vi "Save-Recall State.vi"(0 "VISA resource name":refnum<visa-resource-name>, 1 "saver's name":string, 2 "saved state comments":string, 5 "save/recall (f : recall)":bool, 7 "file name (read description)":path, 11 "error in (no error)":errorcluster, 12 "saved state title":string) -> (3 "recaller's name":string, 4 "VISA resource name out":refnum<visa-resource-name>, 6 "recalled state comments":string, 8 "recalled state date":string, 10 "recalled state time":string, 14 "recalled state title":string, 15 "error out":errorcluster)   [LabVIEW 2018, in "Agilent 87XX Series.lvlib"]
doc: "This VI for the HP8753B Network Analyzer is used for saving instrument states. An instrument state is all the stimulus and response parameters that set up the instrument to make a specific measurement. This information is called the learn string.\n\n The learn string is an encoded array containing only the data need to re-create the state. For example, to re-create a frequency list the HP8753B only needs to save the start frequency, frequency span, and the number of points in each segment. Each point is not recorded. Thus the size of the learn string is not proportional to the number of points in the sweep.\n\n To save calibration data and memory traces you must use the \"save/recall calibration\" and \"save/recall data\" VIs.\n\n When a state is recalled with this VI, the saver's name, the state title, and the save date are written to the instrument display."
uses:
  Agilent 87XX Series.lvlib
panel:
  # "save to file\nrecall from file"
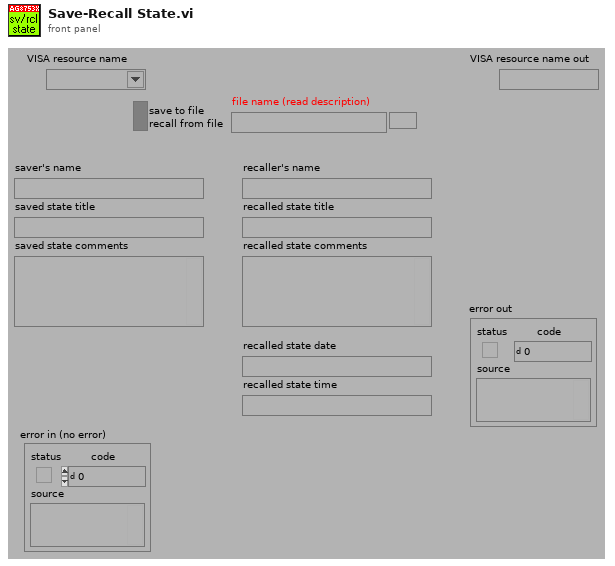
[diagram p1: front panel]
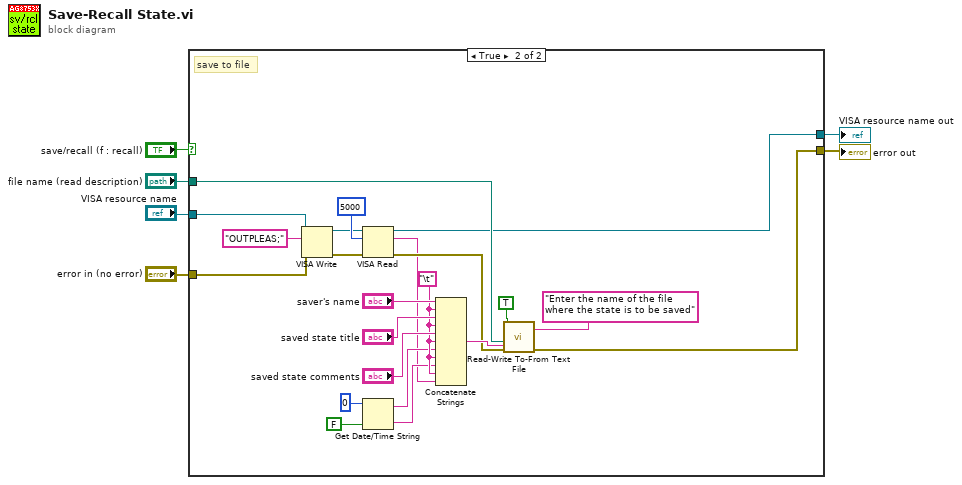
[diagram p0: block diagram]
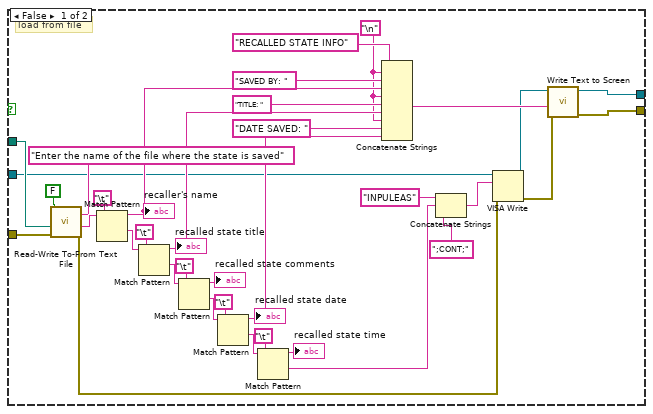
[diagram p2: hidden frame]
diagram:
  n1 = case shown="True" "save/recall (f : recall)" {
    tunnel: "VISA resource name" -> [w16 w50]
    tunnel: "file name (read description)" -> [w20 w51]
    tunnel: "error in (no error)" -> [w15 w49]
    tunnel: [w10 w45] -> w2
    tunnel: [w9 w46] -> w1
    frame False {
      w23 = "\n"
      # "load from file"
      n2 = call "Read-Write To-From Text File.vi"("dialog box prompt"="Enter the name of the file where the state is saved", "error in (no error)"=w15, "file name (read description)"=w20, "read/write (f:read)"=FALSE) -> ("error out"=w14:errorcluster, "string which was read"=w21:string)  [unwired: 6 in]
      n3 = Match Pattern(string=w21, regular expression="\t") -> (before substring=w31:string, after substring=w37:string)  [unwired: 1 in, 2 out]
      "recaller's name" <- w31
      n4 = Match Pattern(string=w37, regular expression="\t") -> (before substring=w28:string, after substring=w36:string)  [unwired: 1 in, 2 out]
      "recalled state title" <- w28
      n5 = Match Pattern(string=w36, regular expression="\t") -> (before substring=→"recalled state comments":string, after substring=w32:string)  [unwired: 1 in, 2 out]
      n6 = Match Pattern(string=w32, regular expression="\t") -> (before substring=w27:string, after substring=w35:string)  [unwired: 1 in, 2 out]
      "recalled state date" <- w27
      n7 = Match Pattern(string=w35, regular expression="\t") -> (before substring=→"recalled state time":string, after substring=w7:string)  [unwired: 1 in, 2 out]
      n8 = Concatenate Strings("RECALLED STATE INFO", w23, "SAVED BY: ", w31, w23, "TITLE: ", w28, w23, "DATE SAVED: ", w27) -> (w13:string)
      n9 = Concatenate Strings("INPULEAS", w7, ";CONT;") -> (w8:string)
      n10 = VISA Write(VISA resource name=w16, write buffer=w8, error in (no error)=w14) -> (VISA resource name out=w12:refnum<visa-resource-name>, error out=w11:errorcluster)  [unwired: 1 out]
      n11 = call "Write Text to Screen.vi"("error in (no error)"=w11, "text"=w13, "VISA session"=w12) -> ("error out"=w9:errorcluster, "dup VISA session"=w10:refnum<visa-resource-name>)  [unwired: 7 in]
    }
    frame True {
      w60 = "\t"
      # "save to file"
      n12 = VISA Write(VISA resource name=w50, write buffer="OUTPLEAS;", error in (no error)=w49) -> (VISA resource name out=w42:refnum<visa-resource-name>, error out=w48:errorcluster)  [unwired: 1 out]
      n13 = VISA Read(VISA resource name=w42, byte count=u32 5000, error in (no error)=w48) -> (VISA resource name out=w45:refnum<visa-resource-name>, read buffer=w44:string, error out=w47:errorcluster)  [unwired: 1 out]
      n14 = Get Date/Time String(date format (0)=0, want seconds? (F)=FALSE) -> (date string=w58:string, time string=w59:string)  [unwired: 1 in]
      n15 = Concatenate Strings("saver's name", w60, "saved state title", w60, "saved state comments", w60, w58, w60, w59, w60, w44) -> (w54:string)
      n16 = call "Read-Write To-From Text File.vi"("string to be written"=w54, "dialog box prompt"="Enter the name of the file where the state is to be saved", "error in (no error)"=w47, "file name (read description)"=w51, "read/write (f:read)"=TRUE) -> ("error out"=w46:errorcluster)  [unwired: 5 in, 1 out]
    }
  }
  "error out" <- w1
  "VISA resource name out" <- w2
